vi "Parse.vi"(8 "Error In":errorcluster, 11 "object in":refnum<class "2021_1.lvclass">) -> (0 "Error Out":errorcluster, 3 "object out":refnum<class "2021_1.lvclass">)   [LabVIEW 2020, in "2021_1.lvclass"]
uses:
  2021_1.lvclass
  2021_1.lvclass/2021_1.ctl
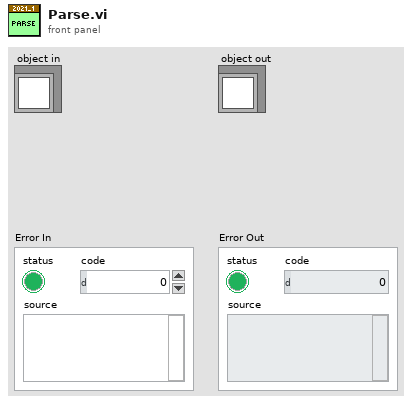
[diagram p1: front panel]
diagram:
  n1 = Spreadsheet String To Array(delimiter (Tab)="\n", format string="%d", spreadsheet string="174\n180\n179\n186\n184\n176\n177\n190\n173\n174\n176\n175\n172\n175\n174\n175\n176\n179\n206\n207\n206\n205\n208\n209\n215\n221\n228\n227\n214\n215\n216\n218\n244\n246\n242\n249\n250\n253\n259\n256\n261\n256\n252\n254\n256\n261\n274\n270\n300\n301\n308\n310\n308\n305\n306\n300\n292\n290\n296\n295\n298\n301\n303\n304\n305\n302\n301\n282\n280\n281\n279\n302\n285\n278\n288\n302\n306\n308\n314\n319\n324\n320\n324\n326\n296\n297\n309\n316\n315\n327\n328\n341\n339\n338\n329\n330\n328\n330\n328\n327\n336\n332\n330\n331\n336\n338\n342\n358\n360\n369\n371\n378\n380\n385\n382\n381\n383\n417\n421\n422\n424\n425\n426\n454\n455\n457\n467\n499\n507\n513\n507\n513\n512\n509\n500\n501\n508\n507\n509\n512\n529\n530\n529\n530\n529\n518\n526\n523\n518\n521\n..." ("PuzzleInput"), array type (2D Dbl)=i32[] []) -> (array=w1:i32[])
  n2 = Bundle By Name(cluster="object in", "Numbers"=w1) -> (→"object out":refnum<class "2021_1.lvclass">)
  "Error Out" <- "Error In"
